vi "oa_XYGraphToWaveform.vi"(0 "input speed profile":T1 {"speed [RPM]" format="%.2f"; "time [s]" format="%.2f"}, 1 "reset? (F)":bool, 5 "analog tacho signal":waveform(dbl)={"t0"=timestamp(0 s since 1904-01-01), "dt"=0.0, "Y"=[]}, 7 "update rate(s)":dbl=0.01, 11 "error in (no error)":errorcluster) -> (4 "speed profile":waveform(dbl), 15 "error out":errorcluster)   [LabVIEW 2017, in "SoundVib_TachProcess.lvlib"]
uses:
  <vilib>/addons/Sound and Vibration/Order Analysis/Tach Process/SoundVib_TachProcess.lvlib
  <vilib>/addons/Sound and Vibration/Order Analysis/Tach Process/SubVIs/speed profile.ctl
  <vilib>/Analysis/1siggen.llb/Ramp Pattern by Samples.vi
  <vilib>/Waveform/WDTOps.llb/WDT Waveform Duration DBL.vi
  <vilib>/Analysis/NI_AALBase.lvlib
panel:
  in  "Waveform":waveform(dbl)={"t0"=timestamp(0 s since 1904-01-01), "dt"=0.0, "Y"=[]}
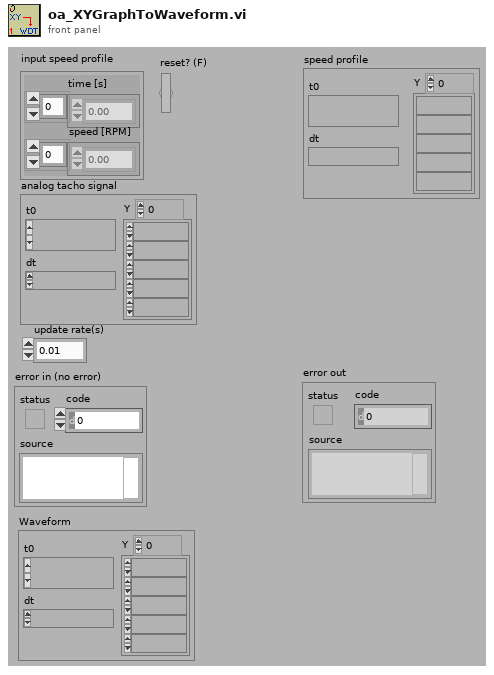
[diagram p1: front panel]
types:
  T1 = typedef "SoundVib_TachProcess.lvlib/speed profile.ctl" = cluster{"time [s]":dbl[], "speed [RPM]":dbl[]}
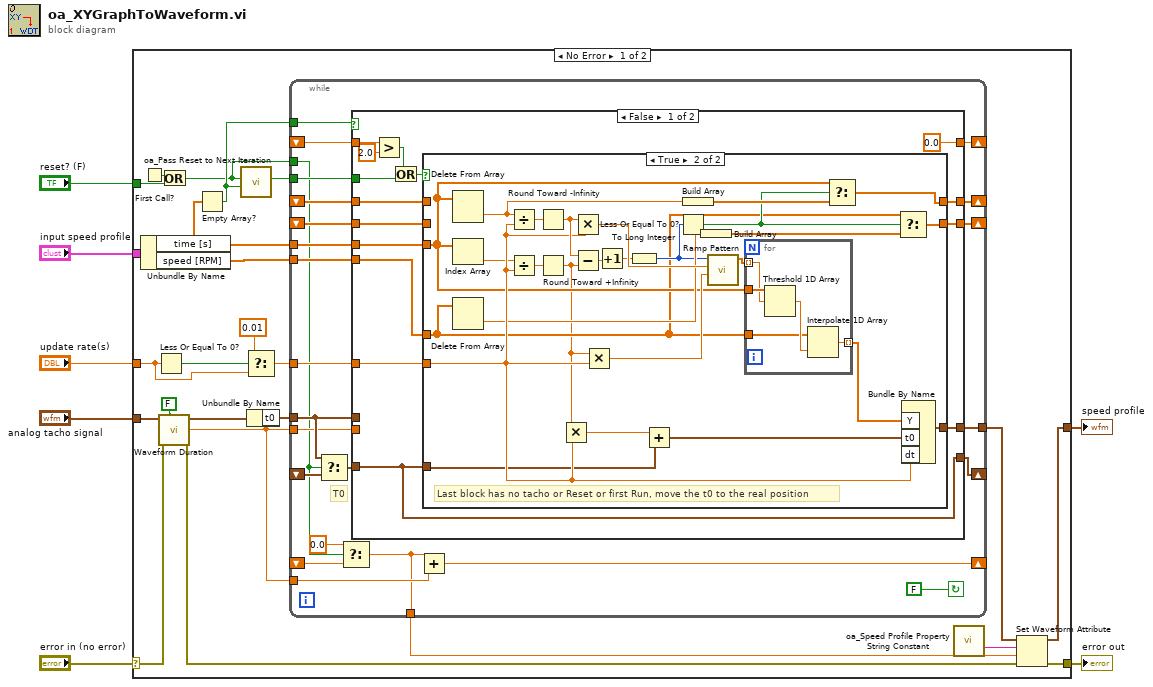
[diagram p0: block diagram]
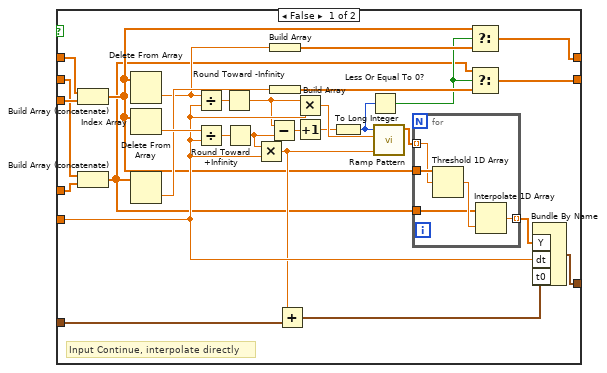
[diagram p2: hidden frame]
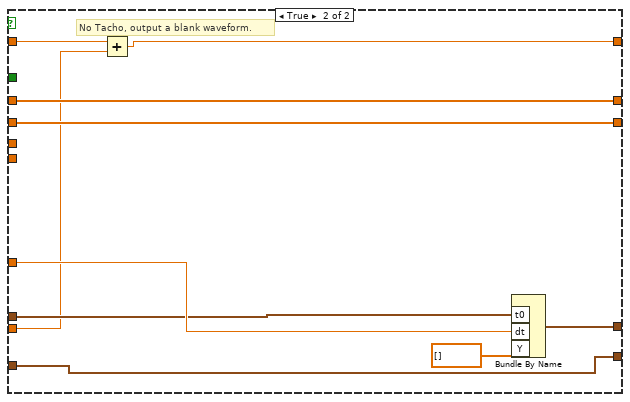
[diagram p3: hidden frame]
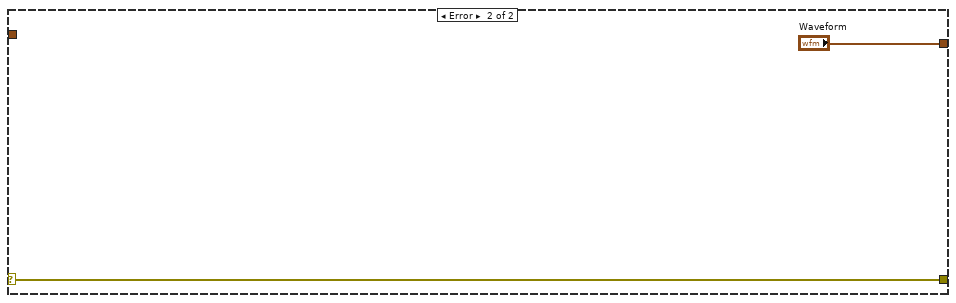
[diagram p4: hidden frame]
diagram:
  n1 = case shown="No Error" "error in (no error)" {
    selector: "error in (no error)" -> [w20 w146]
    tunnel: "reset? (F)" -> [w31 _]
    tunnel: "update rate(s)" -> [w26 _]
    tunnel: [w14 "Waveform"] -> w3
    tunnel: "input speed profile" -> [w29 _]
    tunnel: [w17 w146] -> w4
    tunnel: "analog tacho signal" -> [w21 _]
    frame No Error {
      n2 = First Call?() -> (First Call?: T/F=w30:bool)
      n3 = Unbundle By Name(w29) -> ("time [s]"=w12:dbl[], "speed [RPM]"=w28:dbl[])
      n4 = Less Or Equal To 0?(x=w26) -> (x <= 0?=w27:bool)
      n5 = call-poly <vilib>:"Waveform Duration.vi"("open interval? (T)"=FALSE, "error in (no error)"=w20, "waveform in"=w21) -> ("error out"=w18:errorcluster, "duration"=w13:dbl, "waveform out"=w19:waveform(dbl))  [unwired: 6 in]
      n6 = Or(x=w30, y=w31) -> (x .or. y?=w8:bool)
      n7 = Empty Array?(array=w12) -> (empty?=w9:bool)
      n8 = call <vilib>:"oa_Pass Reset to Next Iteration.vi"("trigger"=w9, "reset?(F)"=w8) -> ("reset out"=w10:bool)  [unwired: 9 in]
      n9 = Select(t=0.01, s=w27, f=w26) -> (s? t:f=w24:dbl)
      n10 = Unbundle By Name(w19) -> ("t0"=w23:timestamp)
      n11 = while {
        tunnel: w10 -> [w33]
        tunnel: w9 -> [w55]
        tunnel: w23 -> [w38]
        tunnel: w24 -> [w54]
        tunnel: [w53] -> w16
        shift-right: [w50] -> _
        shift-left: _ -> [w52]
        tunnel: w12 -> [w49]
        tunnel: w28 -> [w48]
        shift-right: [w47] -> _
        shift-left: _ -> [w45]
        shift-right: [w46] -> _
        shift-left: _ -> [w44]
        shift-right: [w41] -> _
        shift-left: _ -> [w40]
        tunnel: w13 -> [w42]
        tunnel: [w34] -> w15
        shift-right: [w37] -> _
        shift-left: _ -> [w36]
        tunnel: w13 -> [w35]
        tunnel: w8 -> [w32]
        stop <- FALSE continue-if-true
        # "T0"
        n12 = Select(t=w38, s=w32, f=w52) -> (s? t:f=w51:timestamp)
        n13 = Select(t=0.0, s=w32, f=w40) -> (s? t:f=w34:dbl)
        n14 = case shown="False" w55 {
          tunnel: w54 -> [w67 w143]
          tunnel: [w64 w144] -> w53
          tunnel: w51 -> [w68 w139]
          tunnel: [w68 w139] -> w50
          tunnel: w33 -> [w60 _]
          tunnel: w49 -> [w66 _]
          tunnel: w48 -> [w65 _]
          tunnel: [w70 w142] -> w47
          tunnel: [w69 w141] -> w46
          tunnel: w38 -> [_ w140]
          tunnel: w45 -> [w63 w142]
          tunnel: w44 -> [w62 w141]
          tunnel: [0.0 ("deleted portion") w136] -> w37
          tunnel: w36 -> [w58 w138]
          tunnel: w35 -> [_ w137]
          frame False {
            n15 = Greater?(x=w58, y=2.0) -> (0:w57:bool)
            n16 = Or(x=w57, y=w60) -> (x .or. y?=w56:bool)
            n17 = case shown="True" w56 {
              tunnel: [w73 w114] -> w70
              tunnel: [w74 w112] -> w69
              tunnel: w68 -> [w92 w121]
              tunnel: w67 -> [w86 w122]
              tunnel: w66 -> [w99 w108]
              tunnel: w65 -> [w98 w107]
              tunnel: [w87 w124] -> w64
              tunnel: w63 -> [w76 _]
              tunnel: w62 -> [w75 _]
              frame False {
                # "Input Continue, interpolate directly"
                n18 = Build Array (concatenate)(w76, w99) -> (w72:dbl[])
                n19 = Build Array (concatenate)(w75, w98) -> (w71:dbl[])
                n20 = Delete From Array(array=w72) -> (deleted portion=w79:dbl)  [unwired: 2 in, 1 out]
                n21 = Index Array(array=w72) -> (element=w93:dbl)  [unwired: 1 in]
                n22 = Delete From Array(array=w71) -> (deleted portion=w81:dbl)  [unwired: 2 in, 1 out]
                n23 = Divide(x=w79, y=w86) -> (x/y=w97:dbl)
                n24 = Divide(x=w93, y=w86) -> (x/y=w96:dbl)
                n25 = Round Toward -Infinity(1:w97) -> (0:w84:dbl)
                n26 = Round Toward +Infinity(x=w96) -> (ceil(x): smallest int >= x=w90:dbl)
                n27 = Multiply(x=w90, y=w86) -> (x*y=w85:dbl)
                n28 = Subtract(x=w84, y=w90) -> (x-y=w95:dbl)
                n29 = Build Array(w79) -> (w78:dbl[])
                n30 = Build Array(w81) -> (w80:dbl[])
                n31 = Add(x=w85, y=w92) -> (x+y=w88:timestamp)
                n32 = Multiply(x=w84, y=w86) -> (x*y=w94:dbl)
                n33 = Increment(x=w95) -> (x+1=w83:dbl)
                n34 = To Long Integer(number=w83) -> (32bit integer=w82:i32)
                n35 = Less Or Equal To 0?(x=w82) -> (x <= 0?=w77:bool)
                n36 = call-poly <vilib>:"Ramp Pattern.vi"("start"=w85, "end"=w94, "samples"=w82) -> ("Ramp Pattern"=w91:dbl[])  [unwired: 7 in, 1 out]
                n37 = for {
                  tunnel: w91 -> [w103] mode=indexing
                  tunnel: w72 -> [w104]
                  tunnel: w71 -> [w101]
                  tunnel: [w100] -> w89 mode=indexing
                  n38 = Threshold 1D Array(2:w103, 3:w104) -> (0:w102:dbl)  [unwired: 1 in]
                  n39 = Interpolate 1D Array(1:w102, 2:w101) -> (0:w100:dbl)
                }
                n40 = Select(t=w72, s=w77, f=w78) -> (s? t:f=w73:dbl[])
                n41 = Select(t=w71, s=w77, f=w80) -> (s? t:f=w74:dbl[])
                n42 = Bundle By Name("Y"=w89, "dt"=w86, "t0"=w88) -> (w87:waveform(dbl))  [unwired: 1 in]
              }
              frame True {
                # "Last block has no tacho or Reset or first Run, move the t0 to the real position"
                n43 = Delete From Array(array=w108) -> (deleted portion=w116:dbl)  [unwired: 2 in, 1 out]
                n44 = Index Array(array=w108) -> (element=w117:dbl)  [unwired: 1 in]
                n45 = Delete From Array(array=w107) -> (deleted portion=w113:dbl)  [unwired: 2 in, 1 out]
                n46 = Divide(x=w116, y=w122) -> (x/y=w130:dbl)
                n47 = Divide(x=w117, y=w122) -> (x/y=w129:dbl)
                n48 = Round Toward -Infinity(1:w130) -> (0:w123:dbl)
                n49 = Round Toward +Infinity(x=w129) -> (ceil(x): smallest int >= x=w105:dbl)
                n50 = Multiply(x=w105, y=w122) -> (x*y=w120:dbl)
                n51 = Multiply(x=w123, y=w122) -> (x*y=w127:dbl)
                n52 = Subtract(x=w123, y=w105) -> (x-y=w128:dbl)
                n53 = Multiply(x=w105, y=w122) -> (x*y=w126:dbl)
                n54 = Increment(x=w128) -> (x+1=w118:dbl)
                n55 = To Long Integer(number=w118) -> (32bit integer=w110:i32)
                n56 = Add(x=w120, y=w121) -> (x+y=w119:timestamp)
                n57 = Less Or Equal To 0?(x=w110) -> (x <= 0?=w109:bool)
                n58 = Build Array(w116) -> (w115:dbl[])
                n59 = Build Array(w113) -> (w111:dbl[])
                n60 = call-poly <vilib>:"Ramp Pattern.vi"("start"=w126, "end"=w127, "samples"=w110) -> ("Ramp Pattern"=w125:dbl[])  [unwired: 7 in, 1 out]
                n61 = for {
                  tunnel: w125 -> [w134] mode=indexing
                  tunnel: w108 -> [w135]
                  tunnel: w107 -> [w132]
                  tunnel: [w131] -> w106 mode=indexing
                  n62 = Threshold 1D Array(2:w134, 3:w135) -> (0:w133:dbl)  [unwired: 1 in]
                  n63 = Interpolate 1D Array(1:w133, 2:w132) -> (0:w131:dbl)
                }
                n64 = Select(t=w108, s=w109, f=w115) -> (s? t:f=w114:dbl[])
                n65 = Select(t=w107, s=w109, f=w111) -> (s? t:f=w112:dbl[])
                n66 = Bundle By Name("Y"=w106, "t0"=w119, "dt"=w122) -> (w124:waveform(dbl))  [unwired: 1 in]
              }
            }
          }
          frame True {
            # "No Tacho, output a blank waveform."
            n67 = Add(x=w138, y=w137) -> (x+y=w136:dbl)
            n68 = Bundle By Name("t0"=w140, "dt"=w143, "Y"=dbl[] []) -> (w144:waveform(dbl))  [unwired: 1 in]
          }
        }
        n69 = Add(x=w34, y=w42) -> (x+y=w41:dbl)
      }
      n70 = call <vilib>:"oa_Speed Profile Property String Constant.vi"() -> ("elapsed time"=w11:string)  [unwired: 12 in, 3 out]
      n71 = Set Waveform Attribute(4:w18, 5:w15, 6:w11, 7:w16) -> (0:w17:errorcluster, 3:w14:waveform(dbl))  [unwired: 1 out]
    }
    frame Error {
    }
  }
  "error out" <- w4
  "speed profile" <- w3
